vi "Set Resistor copy.vi"(8 "error in":errorcluster, 9 "Set Resistance":T1) -> (0 "error out":errorcluster)   [LabVIEW 2019]
uses:
  <userlib>/LevyLab/Relay Box/Relay-Box.lvclass
  <userlib>/LevyLab/Relay Box/subVIs/Control Relay (256).vi
  <userlib>/LevyLab/Relay Box/Typedefs/Resistor--enum.ctl
panel:
  out "USB":bool
  out "short":bool
  out "0 ohm":bool
  out "100k":bool
  out "10M":bool
  out "Gohm":bool
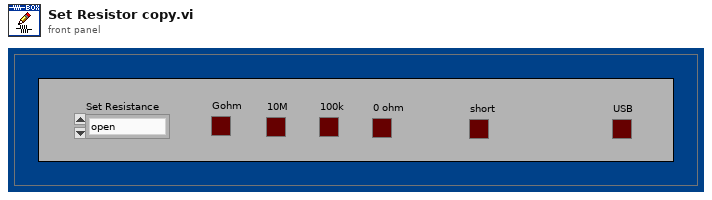
[diagram p1: front panel]
types:
  T1 = typedef "Resistor--enum.ctl" = enum16{"open", "discharge tip", "0 ohms", "100k ohm", "10M ohm", "1G ohm"}
  T2 = enum32{"Invalid", "Standard", "Closed", "Hidden", "Minimized", "Maximized"}
  T3 = enum32{"invalid app kind", "Development System", "Run Time System", "Student Edition", "Embedded LabVIEW", "Evaluation", "Custom"}
  T4 = cluster{"Core":cluster{"Current VI Reference":refnum<vi>, "Close Panel on Exit?":bool}, "Set Resistance":T1, "Previous State":u8, "Intermediate State":u8, "Final State":u8, "Bool Status":bool[]}
  T5 = cluster{"Current VI Reference":refnum<vi>, "Close Panel on Exit?":bool}
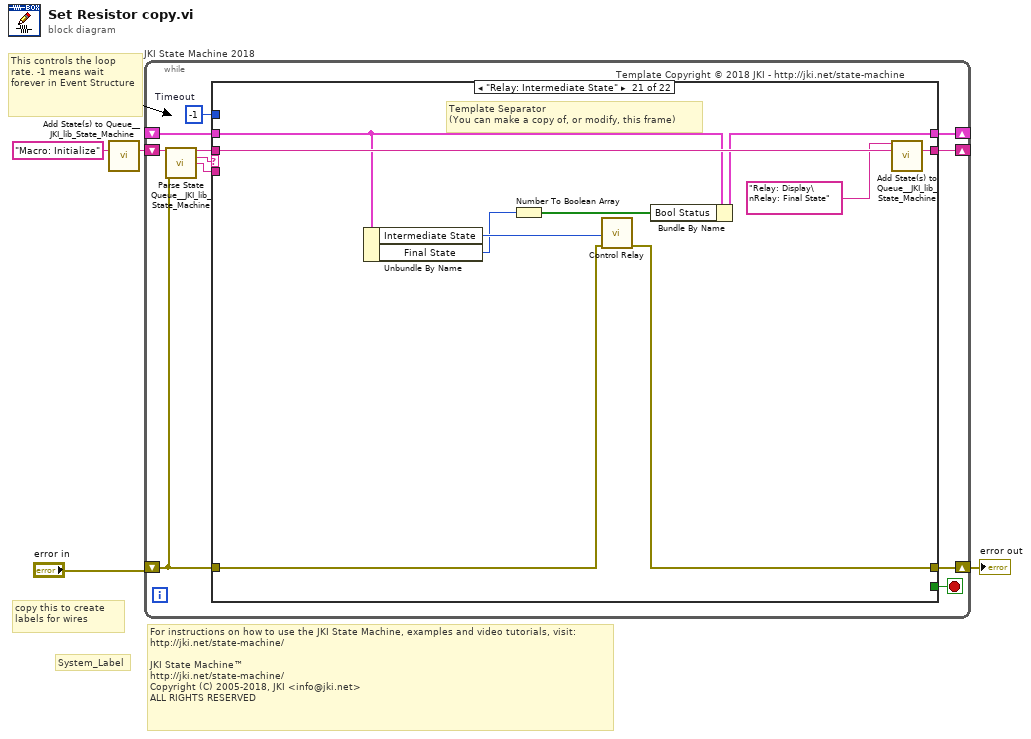
[diagram p0: block diagram]
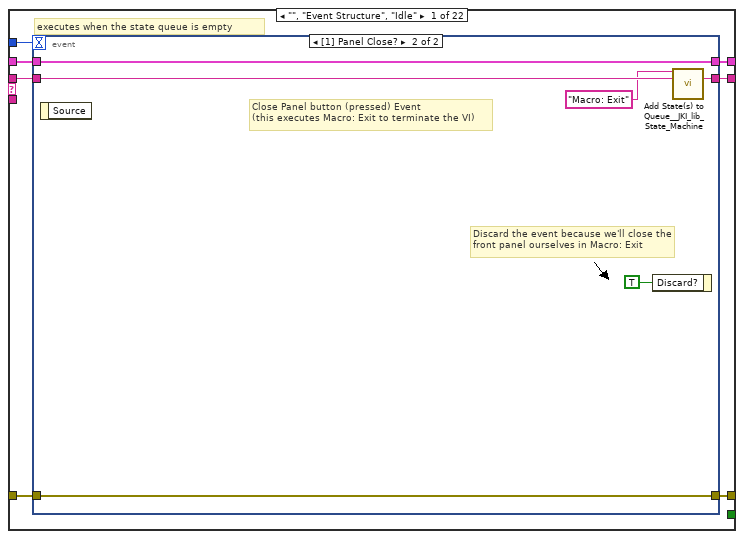
[diagram p2: hidden frame]
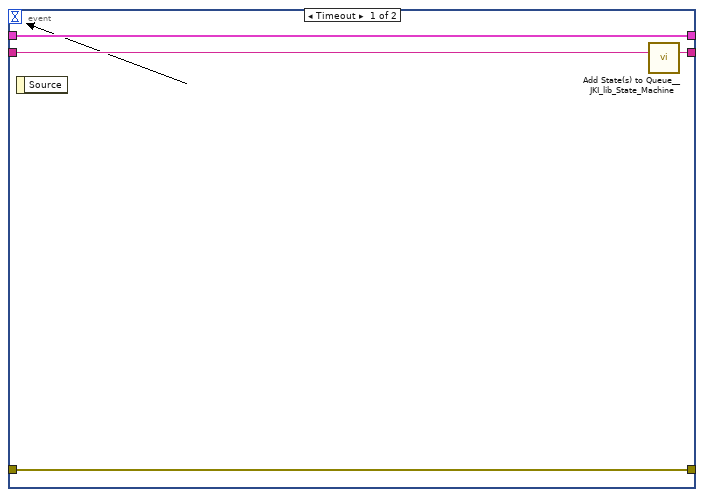
[diagram p3: hidden frame]
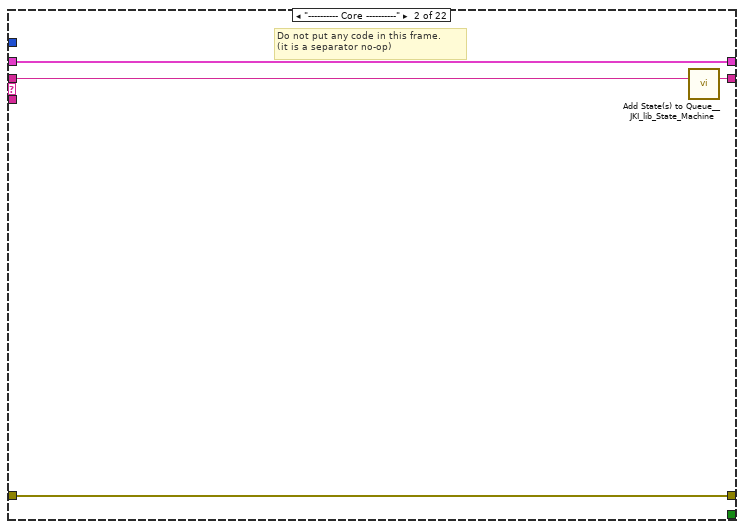
[diagram p4: hidden frame]
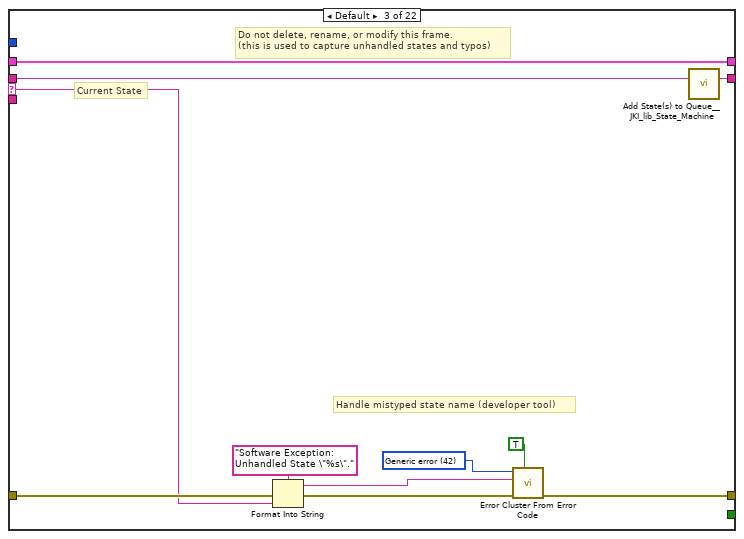
[diagram p5: hidden frame]
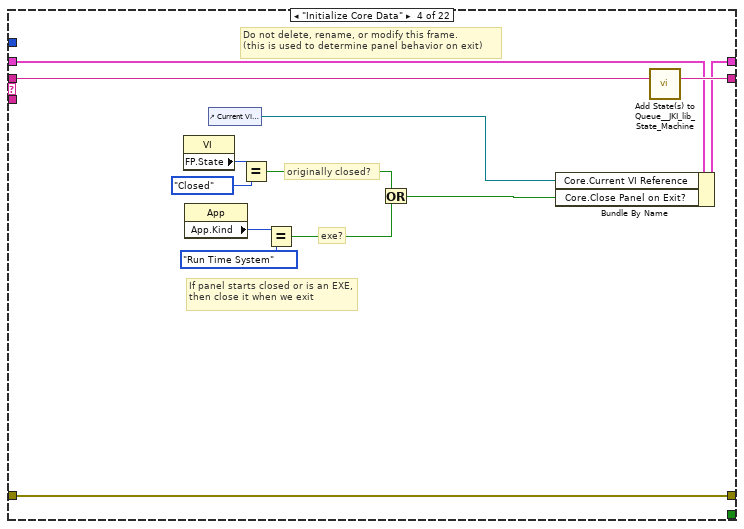
[diagram p6: hidden frame]
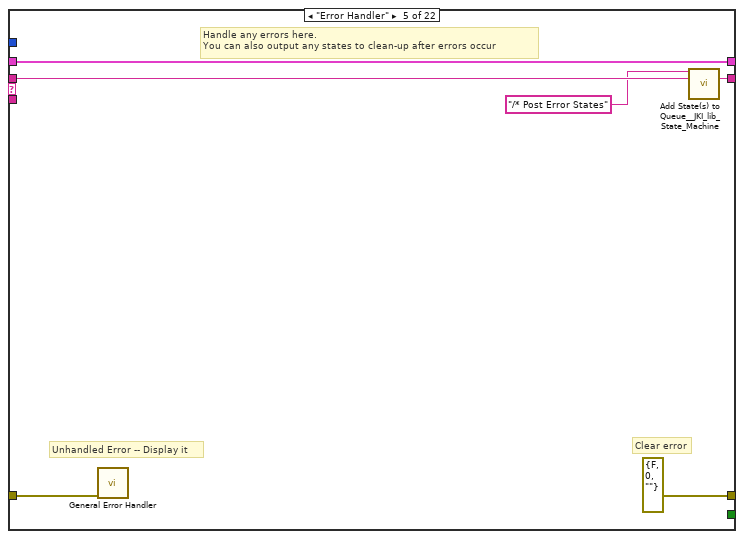
[diagram p7: hidden frame]
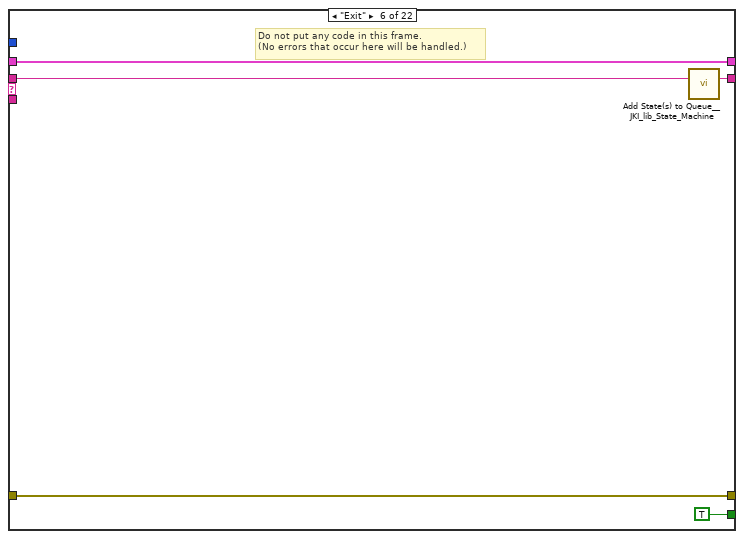
[diagram p8: hidden frame]
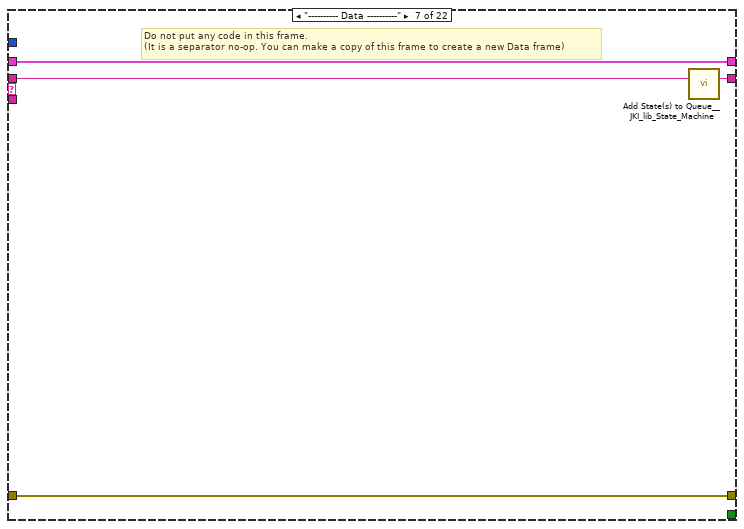
[diagram p9: hidden frame]
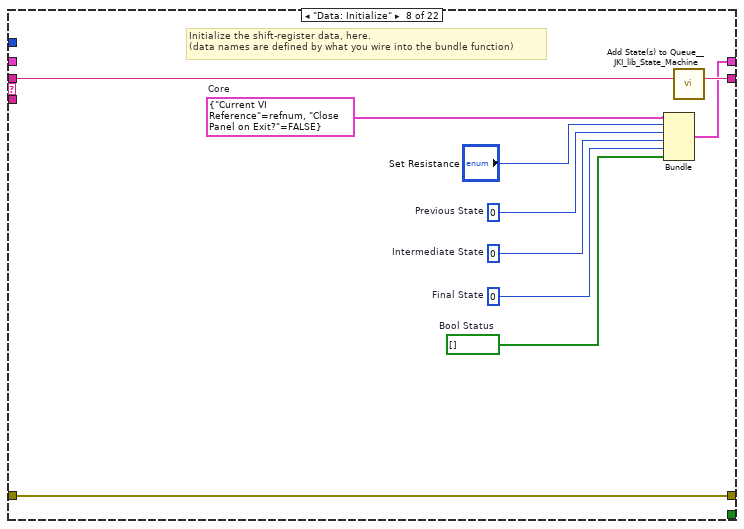
[diagram p10: hidden frame]
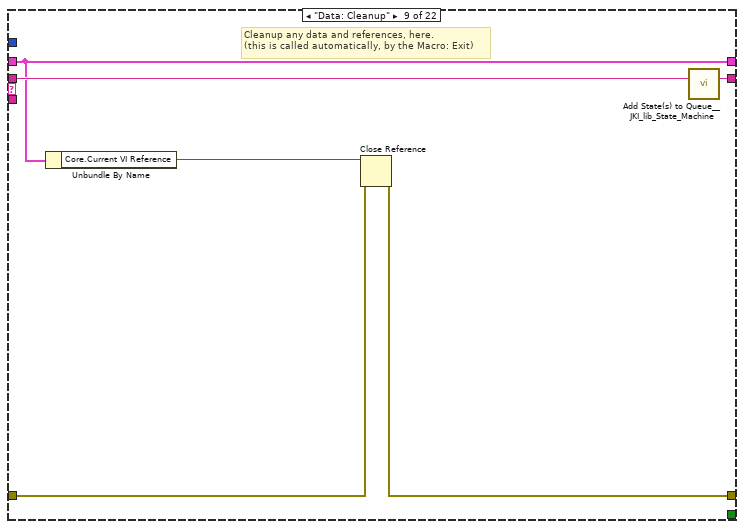
[diagram p11: hidden frame]
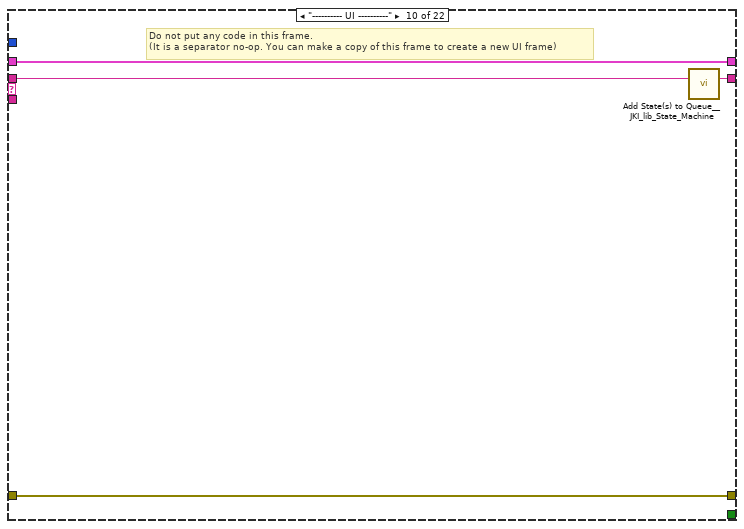
[diagram p12: hidden frame]
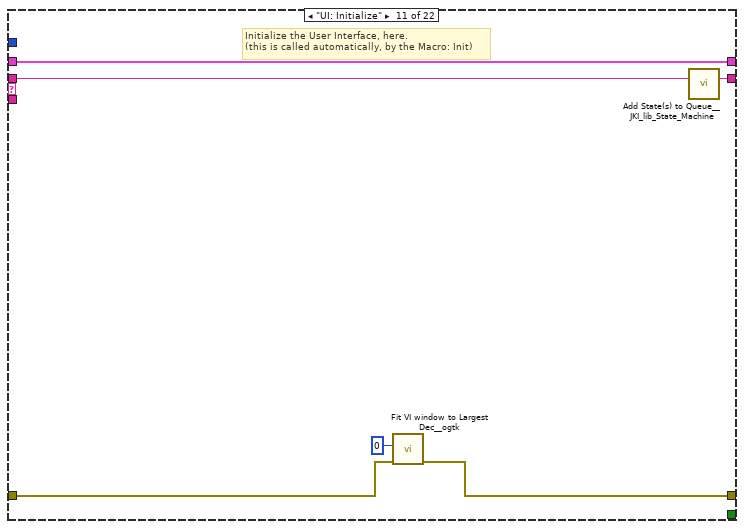
[diagram p13: hidden frame]
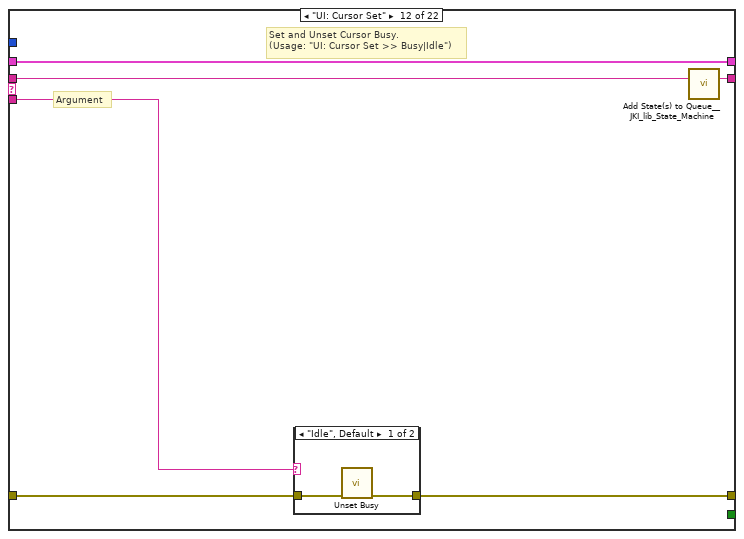
[diagram p14: hidden frame]
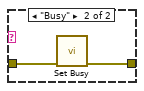
[diagram p15: hidden frame]
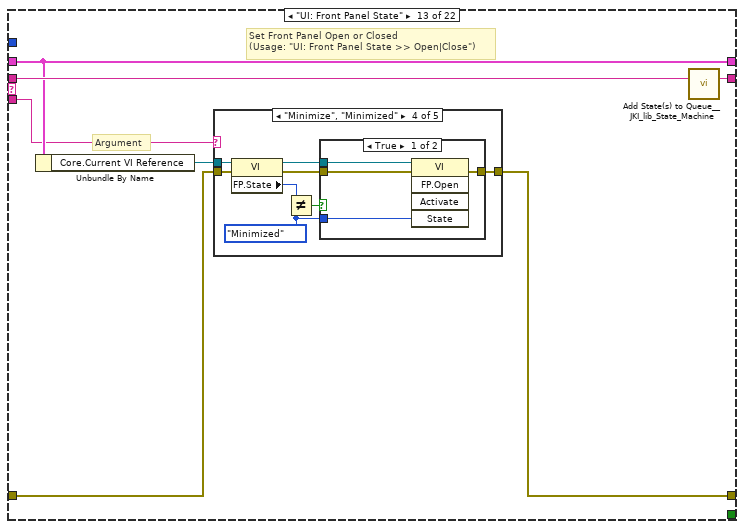
[diagram p16: hidden frame]
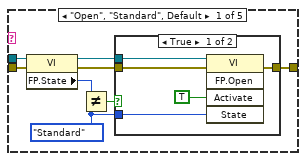
[diagram p17: hidden frame]
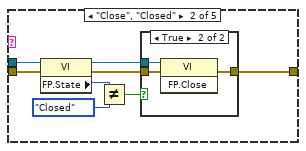
[diagram p19: hidden frame]
diagram:
  # "For instructions on how to use the JKI State Machine, examples and video tutorials, visit:\nhttp://jki.net/state-machine/\n\nJKI State Machine™\nhttp://jki.net/state-machine/\nCopyright (C) 2005-2018, JKI <info@jki.net>\nALL RIGHTS RESERVED"
  # "copy this to create labels for wires"
  # "This controls the loop rate. -1 means wait forever in Event Structure"
  # "System_Label"
  n1 = call <vilib>:"Add State(s) to Queue__JKI_lib_State_Machine.vi"("State(s) in (\"\")"="Macro: Initialize") -> ("States Out"=w4:string)  [unwired: 14 in]
  n2 = while "JKI State Machine 2018" {
    shift-right: [w8] -> _
    shift-left: _ -> [w7]
    shift-right: [w11] -> w2
    shift-left: "error in" -> [w5]
    shift-right: [w10] -> _
    shift-left: w4 -> [w12]
    stop <- w9 stop-if-true
    w6 = -1  # Timeout
    # "Template Copyright © 2018 JKI - http://jki.net/state-machine"
    n3 = call <vilib>:"Parse State Queue__JKI_lib_State_Machine.vi"("State Queue"=w12, "Error In (no error)"=w5) -> ("Remaining States"=w14:string, "Current State"=w15:string, "Arguments"=w13:string)  [unwired: 11 in]
    n4 = case shown="\"Relay: Intermediate State\"" w15 {
      selector: w15 -> [_ _ w37 _ _ _ _ _ _ _ _ _ _ _ _ _ _ _ _ _ _ _]
      tunnel: w14 -> [w22 w36 w41 w60 w66 w71 w75 w85 w91 w95 w101 w107 w118 w187 w192 w202 w206 w222 w230 w244 w368 w375]
      tunnel: w13 -> [_ _ _ _ _ _ _ _ _ _ _ w102 w112 _ _ _ _ _ _ _ _ _]
      tunnel: w7 -> [w20 w33 w39 w53 w63 w69 w72 _ w86 w92 w99 w105 w114 w184 w189 w199 w203 w216 w225 w233 w361 w369]
      tunnel: [w19 w34 w43 w57 errorcluster {"status"=FALSE, "code"=0, "source"=""} ("error out") w68 w73 w83 w87 w93 w97 w103 w115 w185 w190 w200 w204 w220 w228 w242 w362 w371] -> w11
      tunnel: w5 -> [w18 w34 w42 w57 w62 w68 w73 w83 w88 w93 w96 w104 w116 w185 w190 w200 w204 w220 w228 w242 w363 w372]
      tunnel: [w21 w35 w40 w59 w65 w70 w74 w84 w90 w94 w100 w106 w117 w186 w191 w201 w205 w221 w229 w243 w367 w374] -> w10
      tunnel: [_ _ _ _ _ TRUE _ _ _ _ _ _ _ _ _ _ _ _ _ _ _ _] -> w9
      tunnel: [w17 w33 w39 w58 w63 w69 w72 w77 w86 w92 w99 w105 w114 w184 w189 w199 w203 w216 w224 w232 w360 w369] -> w8
      tunnel: w6 -> [w16 _ _ _ _ _ _ _ _ _ _ _ _ _ _ _ _ _ _ _ _ _]
      frame "", "Event Structure", "Idle" {
        # "executes when the state queue is empty"
        n5 = event shown="[1] Panel Close?" {
          selector: _ -> [_ _]
          dyn-events: _ -> [_ _]
          timeout: w16 -> [_ _]
          tunnel: w22 -> [w26 w32]
          tunnel: [w25 w31] -> w21
          tunnel: w20 -> [w23 w29]
          tunnel: [w24 w30] -> w19
          tunnel: w18 -> [w24 w30]
          tunnel: [w23 w29] -> w17
          event Timeout {
            n6 = event-data() -> ()  [unwired: 1 in, 1 out]
            n7 = call <vilib>:"Add State(s) to Queue__JKI_lib_State_Machine.vi"("State(s) in (\"\")"=w26) -> ("States Out"=w25:string)  [unwired: 14 in]
          }
          event Panel Close? {
            # "Discard the event because we'll close the front panel ourselves in Macro: Exit"
            # "Close Panel button (pressed) Event\n(this executes Macro: Exit to terminate the VI)"
            n8 = event-data() -> ()  [unwired: 1 in, 1 out]
            n9 = event-data("Discard?"=TRUE) -> ()  [unwired: 1 in, 1 out]
            n10 = call <vilib>:"Add State(s) to Queue__JKI_lib_State_Machine.vi"("State(s) in Front (\"\")"="Macro: Exit", "State(s) in (\"\")"=w32) -> ("States Out"=w31:string)  [unwired: 13 in]
          }
        }
      }
      frame "---------- Core ----------" {
        # "Do not put any code in this frame.\n(it is a separator no-op)"
        n11 = call <vilib>:"Add State(s) to Queue__JKI_lib_State_Machine.vi"("State(s) in (\"\")"=w36) -> ("States Out"=w35:string)  [unwired: 14 in]
      }
      frame Default {
        w46 = 42 items=["No error", "Argument error", "Memory is full", "Out of zone", "End of file", "File already open", "Generic file I/O error", "File not found", "File permission error", "Disk is full", "Duplicate path", "Too many files open", "System feature not enabled", "Resource file not found", "Cannot add resource", "Resource not found", "Image not found", "Image memory error", "Pen does not exist", "Config type invalid", "Config token not found", "Config parse error", "Config memory error", "Bad external code format", "Bad external code offset", "External code not present", "Null window", "Destroy window error", "Null menu", "Print aborted", "Bad print record", "Print driver error", "Windows error during printing", "Memory error during printing", "Print dialog error", "Generic print error", "Invalid device refnum", "Device not found", "Device parameter error", "Device unit error", "Cannot open device", "Device call aborted", "Generic error", "Cancelled by user", "Object ID too low", "Object ID too high", "Object not in heap", "Unknown heap", "Unknown object (invalid DefProc)", "Unknown object (DefProc not in table)", "Message out of range", "Invalid (null) method", "Unknown message", "Manager call not supported", "Bad address", "Network operation in progress", "Network operation timed out", "Connection is busy", "Network attribute not supported", "Network error", "Address in use", "System out of memory", "Connection aborted", "Connection refused", "Not connected", "Already connected", "Connection closed", "Initialization error (interapplication manager)", "Bad occurrence", "Wait on unbound occurrence handler", "Occurrence queue overflow", "Datalog type conflict", "Unused", "Unrecognized type (interapplication manager)", "Memory corrupt", "Failed to make temporary DLL", "Old CIN version", "Drag socket not found", "Failed to load drop-object", "Failed to register OLE object", "Failed to release OLE object", "Format specifier type mismatch", "Unknown format specifier", "Too few format specifiers", "Too many format specifiers", "Scan failed", "Newer CIN version", "Error converting to variant", "Runtime menu error", "Password tampered", "Variant attribute not found", "Incompatible variant data type", "Event data is not available", "Event Store is not present", "Occurrence is not found", "Event Queue is not created", "Event info is not available", "Refnum passed is NULL", "Error retrieving Class GUID", "Error retrieving CoClass GUID", "Error retrieving TypeLib GUID.", "Bad built application magic bytes.", "Specific driver is different from the specific driver associated with the Logical Name.", "There is no session opened to the class driver.", "Max Error", "MAX - Error with config objects", "MAX - Error loading configuration", "MAX - Group not supported"]
        # "Current State"
        # "Do not delete, rename, or modify this frame.\n(this is used to capture unhandled states and typos)"
        # "Handle mistyped state name (developer tool)"
        n12 = Format Into String(format string="Software Exception: Unhandled State \"%s\"." ("message"), error in=w42, w37) -> (resulting string=w45:string, error out=w44:errorcluster)  [unwired: 1 in]
        n13 = call <vilib>:"Error Cluster From Error Code.vi"("show call chain? (False)"=TRUE, "error in (no error)"=w44, "error message (\"\")"=w45, "error code (0)"=w46) -> ("error out"=w43:errorcluster)  [unwired: 5 in]
        n14 = call <vilib>:"Add State(s) to Queue__JKI_lib_State_Machine.vi"("State(s) in (\"\")"=w41) -> ("States Out"=w40:string)  [unwired: 14 in]
      }
      frame "Initialize Core Data" {
        # "Do not delete, rename, or modify this frame.\n(this is used to determine panel behavior on exit)"
        # "originally closed?"
        # "exe?"
        # "If panel starts closed or is an EXE, then close it when we exit"
        n15 = property class="VI"() -> ("FP.State"=w50:T2)  [unwired: 2 in, 2 out]
        n16 = property class="App"() -> ("App.Kind"=w56:T3)  [unwired: 2 in, 2 out]
        n17 = control-ref of="Current VI Reference"() -> (w51:refnum<vi>)
        n18 = Equal?(x=w50, y=T2."Closed" ("Front Panel Window:State")) -> (x = y?=w48:bool)
        n19 = Equal?(x=w56, y=T3."Run Time System" ("Application:Kind")) -> (x = y?=w54:bool)
        n20 = Or(x=w48, y=w54) -> (x .or. y?=w52:bool)
        n21 = Bundle By Name(cluster=w53, "Core.Current VI Reference"=w51, "Core.Close Panel on Exit?"=w52) -> (w58:T4)
        n22 = call <vilib>:"Add State(s) to Queue__JKI_lib_State_Machine.vi"("State(s) in (\"\")"=w60) -> ("States Out"=w59:string)  [unwired: 14 in]
      }
      frame "Error Handler" {
        # "Unhandled Error -- Display it"
        # "Handle any errors here.\nYou can also output any states to clean-up after errors occur"
        # "Clear error"
        n23 = call <vilib>:"General Error Handler.vi"("error in (no error)"=w62) -> ()  [unwired: 10 in, 5 out]
        n24 = call <vilib>:"Add State(s) to Queue__JKI_lib_State_Machine.vi"("State(s) in Front (\"\")"="/* Post Error States", "State(s) in (\"\")"=w66) -> ("States Out"=w65:string)  [unwired: 13 in]
      }
      frame "Exit" {
        # "Do not put any code in this frame.\n(No errors that occur here will be handled.)"
        n25 = call <vilib>:"Add State(s) to Queue__JKI_lib_State_Machine.vi"("State(s) in (\"\")"=w71) -> ("States Out"=w70:string)  [unwired: 14 in]
      }
      frame "---------- Data ----------" {
        # "Do not put any code in this frame.\n(It is a separator no-op. You can make a copy of this frame to create a new Data frame)"
        n26 = call <vilib>:"Add State(s) to Queue__JKI_lib_State_Machine.vi"("State(s) in (\"\")"=w75) -> ("States Out"=w74:string)  [unwired: 14 in]
      }
      frame "Data: Initialize" {
        w76 = bool[] []  # Bool Status
        w79 = u8 0  # Final State
        w80 = u8 0  # Intermediate State
        w81 = u8 0  # Previous State
        w78 = T5 {"Current VI Reference"=refnum, "Close Panel on Exit?"=FALSE}  # Core
        # "Initialize the shift-register data, here.\n(data names are defined by what you wire into the bundle function)"
        n27 = Bundle("Core"=w78, "Set Resistance"="Set Resistance", "Previous State"=w81, "Intermediate State"=w80, "Final State"=w79, "Bool Status"=w76) -> (w77:T4)  [unwired: 1 in]
        n28 = call <vilib>:"Add State(s) to Queue__JKI_lib_State_Machine.vi"("State(s) in (\"\")"=w85) -> ("States Out"=w84:string)  [unwired: 14 in]
      }
      frame "Data: Cleanup" {
        # "Cleanup any data and references, here.\n(this is called automatically, by the Macro: Exit)"
        n29 = Unbundle By Name(w86) -> ("Core.Current VI Reference"=w89:refnum<vi>)
        n30 = Close Reference(reference=w89, error in (no error)=w88) -> (error out=w87:errorcluster)
        n31 = call <vilib>:"Add State(s) to Queue__JKI_lib_State_Machine.vi"("State(s) in (\"\")"=w91) -> ("States Out"=w90:string)  [unwired: 14 in]
      }
      frame "---------- UI ----------" {
        # "Do not put any code in this frame.\n(It is a separator no-op. You can make a copy of this frame to create a new UI frame)"
        n32 = call <vilib>:"Add State(s) to Queue__JKI_lib_State_Machine.vi"("State(s) in (\"\")"=w95) -> ("States Out"=w94:string)  [unwired: 14 in]
      }
      frame "UI: Initialize" {
        # "Initialize the User Interface, here.\n(this is called automatically, by the Macro: Init)"
        n33 = call <userlib>:"Fit VI window to Largest Dec__ogtk.vi"("error in (no error)"=w96, "border spacing (2 px)"=0) -> ("error out"=w97:errorcluster)  [unwired: 4 in, 1 out]
        n34 = call <vilib>:"Add State(s) to Queue__JKI_lib_State_Machine.vi"("State(s) in (\"\")"=w101) -> ("States Out"=w100:string)  [unwired: 14 in]
      }
      frame "UI: Cursor Set" {
        # "Argument"
        # "Set and Unset Cursor Busy.\n(Usage: \"UI: Cursor Set >> Busy|Idle\")"
        n35 = case shown="\"Idle\", Default" w102 {
          tunnel: w104 -> [w109 w111]
          tunnel: [w108 w110] -> w103
          frame "Idle", Default {
            n36 = call <vilib>:"Unset Busy.vi"("error in (no error)"=w109) -> ("error out"=w108:errorcluster)  [unwired: 10 in]
          }
          frame "Busy" {
            n37 = call <vilib>:"Set Busy.vi"("error in (no error)"=w111) -> ("error out"=w110:errorcluster)  [unwired: 9 in, 1 out]
          }
        }
        n38 = call <vilib>:"Add State(s) to Queue__JKI_lib_State_Machine.vi"("State(s) in (\"\")"=w107) -> ("States Out"=w106:string)  [unwired: 14 in]
      }
      frame "UI: Front Panel State" {
        # "Argument"
        # "Set Front Panel Open or Closed\n(Usage: \"UI: Front Panel State >> Open|Close\")"
        n39 = Unbundle By Name(w114) -> ("Core.Current VI Reference"=w113:refnum<vi>)
        n40 = case shown="\"Minimize\", \"Minimized\"" w112 {
          tunnel: w116 -> [w124 w139 w150 w163 w176]
          tunnel: [w126 w140 w152 w165 w178] -> w115
          tunnel: w113 -> [w125 w137 w151 w164 w177]
          frame "Open", "Standard", Default {
            w119 = T2."Standard" ("State")
            n41 = property class="VI"(reference=w125, error in=w124) -> (reference out=w122:refnum<vi>, error out=w123:errorcluster, "FP.State"=w121:T2)
            n42 = Not Equal?(x=w121, y=w119) -> (x != y?=w120:bool)
            n43 = case shown="True" w120 {
              tunnel: [w130 w132] -> w126
              tunnel: w123 -> [w129 w132]
              tunnel: w122 -> [w128 _]
              tunnel: w119 -> [w127 _]
              frame True {
                n44 = invoke class="VI" method="FP.Open"(reference=w128, error in=w129, "Activate"=TRUE, "State"=w127) -> (error out=w130:errorcluster)  [unwired: 1 in, 4 out]
              }
              frame False {
              }
            }
          }
          frame "Close", "Closed" {
            n45 = property class="VI"(reference=w137, error in=w139) -> (reference out=w136:refnum<vi>, error out=w138:errorcluster, "FP.State"=w134:T2)
            n46 = Not Equal?(x=w134, y=T2."Closed" ("Front Panel Window:State")) -> (x != y?=w133:bool)
            n47 = case shown="True" w133 {
              tunnel: [w141 w144] -> w140
              tunnel: w138 -> [w141 w143]
              tunnel: w136 -> [_ w142]
              frame False {
              }
              frame True {
                n48 = invoke class="VI" method="FP.Close"(reference=w142, error in=w143) -> (error out=w144:errorcluster)  [unwired: 1 in, 2 out]
              }
            }
          }
          frame "Hidden", "Hide" {
            w145 = T2."Hidden" ("State")
            n49 = property class="VI"(reference=w151, error in=w150) -> (reference out=w148:refnum<vi>, error out=w149:errorcluster, "FP.State"=w147:T2)
            n50 = Not Equal?(x=w147, y=w145) -> (x != y?=w146:bool)
            n51 = case shown="True" w146 {
              tunnel: [w156 w157] -> w152
              tunnel: w149 -> [w155 w157]
              tunnel: w148 -> [w154 _]
              tunnel: w145 -> [w153 _]
              frame True {
                n52 = invoke class="VI" method="FP.Open"(reference=w154, error in=w155, "State"=w153) -> (error out=w156:errorcluster)  [unwired: 2 in, 4 out]
              }
              frame False {
              }
            }
          }
          frame "Minimize", "Minimized" {
            w158 = T2."Minimized" ("State")
            n53 = property class="VI"(reference=w164, error in=w163) -> (reference out=w161:refnum<vi>, error out=w162:errorcluster, "FP.State"=w160:T2)
            n54 = Not Equal?(x=w160, y=w158) -> (x != y?=w159:bool)
            n55 = case shown="True" w159 {
              tunnel: [w169 w170] -> w165
              tunnel: w162 -> [w168 w170]
              tunnel: w161 -> [w167 _]
              tunnel: w158 -> [w166 _]
              frame True {
                n56 = invoke class="VI" method="FP.Open"(reference=w167, error in=w168, "State"=w166) -> (error out=w169:errorcluster)  [unwired: 2 in, 4 out]
              }
              frame False {
              }
            }
          }
          frame "Maximize", "Maximized" {
            w171 = T2."Maximized" ("State")
            n57 = property class="VI"(reference=w177, error in=w176) -> (reference out=w174:refnum<vi>, error out=w175:errorcluster, "FP.State"=w173:T2)
            n58 = Not Equal?(x=w173, y=w171) -> (x != y?=w172:bool)
            n59 = case shown="True" w172 {
              tunnel: [w182 w183] -> w178
              tunnel: w175 -> [w181 w183]
              tunnel: w174 -> [w180 _]
              tunnel: w171 -> [w179 _]
              frame True {
                n60 = invoke class="VI" method="FP.Open"(reference=w180, error in=w181, "State"=w179) -> (error out=w182:errorcluster)  [unwired: 2 in, 4 out]
              }
              frame False {
              }
            }
          }
        }
        n61 = call <vilib>:"Add State(s) to Queue__JKI_lib_State_Machine.vi"("State(s) in (\"\")"=w118) -> ("States Out"=w117:string)  [unwired: 14 in]
      }
      frame "---------- Macro ----------" {
        # "Do not put any code in this frame.\n(It is a separator no-op. You can make a copy of this frame to create a new Macro frame)"
        n62 = call <vilib>:"Add State(s) to Queue__JKI_lib_State_Machine.vi"("State(s) in (\"\")"=w187) -> ("States Out"=w186:string)  [unwired: 14 in]
      }
      frame "Macro: Initialize" {
        # "Initialization Macro\n(This is called once, when the VI starts)"
        n63 = call <vilib>:"Add State(s) to Queue__JKI_lib_State_Machine.vi"("State(s) in Front (\"\")"="Data: Initialize\nInitialize Core Data\nUI: Initialize\nRelay: Read\nRelay: Do Logic", "State(s) in (\"\")"=w192) -> ("States Out"=w191:string)  [unwired: 13 in]
      }
      frame "Macro: Exit" {
        # "Exit Macro\n(This is called once, when the VI exits)"
        n64 = Unbundle By Name(w199) -> ("Core.Close Panel on Exit?"=w198:bool)
        n65 = Select(t="UI: Front Panel State >> Close", s=w198, f="") -> (s? t:f=w195:string)
        n66 = call <vilib>:"Add State(s) to Queue__JKI_lib_State_Machine.vi"("State(s) in (\"\")"=w195, "State(s) at Back (\"\")"="Data: Cleanup\nExit") -> ("States Out"=w193:string)  [unwired: 13 in]
        n67 = call <vilib>:"Add State(s) to Queue__JKI_lib_State_Machine.vi"("State(s) in Front (\"\")"=w193, "State(s) in (\"\")"=w202) -> ("States Out"=w201:string)  [unwired: 13 in]
      }
      frame "---------- Relay ----------" {
        # "Template Separator\n(You can make a copy of, or modify, this frame)"
        n68 = call <vilib>:"Add State(s) to Queue__JKI_lib_State_Machine.vi"("State(s) in (\"\")"=w206) -> ("States Out"=w205:string)  [unwired: 14 in]
      }
      frame "Relay: Display" {
        # "Your code here.\n(You can make a copy of, or modify, this frame)"
        n69 = Unbundle By Name(w216) -> ("Bool Status"=w215:bool[])
        n70 = Index Array(array=w215, index #1=7 ("index"), index #2=6 ("index"), index #3=5 ("index"), index #4=3 ("index"), index #5=1 ("index")) -> (element #1=→"Gohm":bool, element #2=→"10M":bool, element #3=→"100k":bool, element #4=→"0 ohm":bool, element #5=→"short":bool)
        n71 = call <vilib>:"Add State(s) to Queue__JKI_lib_State_Machine.vi"("State(s) in (\"\")"=w222) -> ("States Out"=w221:string)  [unwired: 14 in]
        "USB" <- TRUE ("USB")
      }
      frame "Relay: Read" {
        # "Your code here.\n(You can make a copy of, or modify, this frame)"
        n72 = call <userlib>:"Read Relay.vi"() -> ("unsigned 8bit integer"=w227:u8, "Boolean array"=w226:bool[])  [unwired: 1 in]
        n73 = Bundle By Name(cluster=w225, "Previous State"=w227, "Bool Status"=w226) -> (w224:T4)
        n74 = call <vilib>:"Add State(s) to Queue__JKI_lib_State_Machine.vi"("State(s) in Front (\"\")"="Relay: Display" ("State(s) in Front (\"\")"), "State(s) in (\"\")"=w230) -> ("States Out"=w229:string)  [unwired: 13 in]
      }
      frame "Relay: Do Logic" {
        # "Template Separator\n(You can make a copy of, or modify, this frame)"
        n75 = Unbundle By Name(w233) -> ("Set Resistance"=w241:T1, "Previous State"=w237:u8)
        n76 = case shown="\"0 ohms\"" w241 {
          tunnel: [u8 0 w248 w256 w282 w308 w334] -> w236
          tunnel: [FALSE w249 w255 w281 w307 w333] -> w231
          tunnel: [0 2 8 32 64 128] -> w238
          tunnel: w237 -> [_ w251 w257 w283 w309 w335]
          frame "open", Default {
          }
          frame "discharge tip" {
            n77 = Not Equal?(x=w251, y=u8 0) -> (x != y?=w249:bool)
            n78 = case shown="True" w249 {
              tunnel: [u8 2 u8 0] -> w248
              frame False {
              }
              frame True {
              }
            }
          }
          frame "0 ohms" {
            n79 = Not Equal?(x=w257, y=u8 2) -> (x != y?=w258:bool)
            n80 = case shown="True" w258 {
              tunnel: w257 -> [_ w265]
              tunnel: [u8 0 w264] -> w256
              tunnel: [TRUE w263] -> w255
              frame False {
              }
              frame True {
                n81 = Not Equal?(x=w265, y=u8 0) -> (x != y?=w266:bool)
                n82 = case shown="True" w266 {
                  tunnel: w265 -> [_ w273]
                  tunnel: [u8 8 w271] -> w264
                  tunnel: [FALSE w270] -> w263
                  frame False {
                  }
                  frame True {
                    w272 = u8 8 ("y")
                    n83 = Not Equal?(x=w273, y=w272) -> (x != y?=w274:bool)
                    n84 = case shown="False" w274 {
                      tunnel: w273 -> [_ w280]
                      tunnel: w272 -> [_ w279]
                      tunnel: [u8 8 w278] -> w271
                      tunnel: [FALSE TRUE] -> w270
                      frame False {
                      }
                      frame True {
                        n85 = Add(x=w280, y=w279) -> (x+y=w278:u8)
                      }
                    }
                  }
                }
              }
            }
          }
          frame "100k ohm" {
            n86 = Not Equal?(x=w283, y=u8 2) -> (x != y?=w284:bool)
            n87 = case shown="True" w284 {
              tunnel: w283 -> [_ w291]
              tunnel: [u8 0 w290] -> w282
              tunnel: [TRUE w289] -> w281
              frame False {
              }
              frame True {
                n88 = Not Equal?(x=w291, y=u8 0) -> (x != y?=w292:bool)
                n89 = case shown="False" w292 {
                  tunnel: w291 -> [_ w299]
                  tunnel: [u8 32 w297] -> w290
                  tunnel: [FALSE w296] -> w289
                  frame False {
                  }
                  frame True {
                    w298 = u8 32 ("y")
                    n90 = Not Equal?(x=w299, y=w298) -> (x != y?=w300:bool)
                    n91 = case shown="True" w300 {
                      tunnel: w299 -> [_ w306]
                      tunnel: w298 -> [_ w305]
                      tunnel: [u8 32 w304] -> w297
                      tunnel: [FALSE TRUE] -> w296
                      frame False {
                      }
                      frame True {
                        n92 = Add(x=w306, y=w305) -> (x+y=w304:u8)
                      }
                    }
                  }
                }
              }
            }
          }
          frame "10M ohm" {
            n93 = Not Equal?(x=w309, y=u8 2) -> (x != y?=w310:bool)
            n94 = case shown="True" w310 {
              tunnel: w309 -> [_ w317]
              tunnel: [u8 0 w316] -> w308
              tunnel: [TRUE w315] -> w307
              frame False {
              }
              frame True {
                n95 = Not Equal?(x=w317, y=u8 0) -> (x != y?=w318:bool)
                n96 = case shown="False" w318 {
                  tunnel: w317 -> [_ w325]
                  tunnel: [u8 64 w323] -> w316
                  tunnel: [FALSE w322] -> w315
                  frame False {
                  }
                  frame True {
                    w324 = u8 64 ("y")
                    n97 = Not Equal?(x=w325, y=w324) -> (x != y?=w326:bool)
                    n98 = case shown="False" w326 {
                      tunnel: w325 -> [_ w332]
                      tunnel: w324 -> [_ w331]
                      tunnel: [u8 64 w330] -> w323
                      tunnel: [FALSE TRUE] -> w322
                      frame False {
                      }
                      frame True {
                        n99 = Add(x=w332, y=w331) -> (x+y=w330:u8)
                      }
                    }
                  }
                }
              }
            }
          }
          frame "1G ohm" {
            n100 = Not Equal?(x=w335, y=u8 2) -> (x != y?=w336:bool)
            n101 = case shown="True" w336 {
              tunnel: w335 -> [_ w343]
              tunnel: [u8 0 w342] -> w334
              tunnel: [TRUE w341] -> w333
              frame False {
              }
              frame True {
                n102 = Not Equal?(x=w343, y=u8 0) -> (x != y?=w344:bool)
                n103 = case shown="False" w344 {
                  tunnel: w343 -> [_ w351]
                  tunnel: [u8 128 w349] -> w342
                  tunnel: [FALSE w348] -> w341
                  frame False {
                  }
                  frame True {
                    w350 = u8 128 ("y")
                    n104 = Not Equal?(x=w351, y=w350) -> (x != y?=w352:bool)
                    n105 = case shown="True" w352 {
                      tunnel: w351 -> [_ w358]
                      tunnel: w350 -> [_ w357]
                      tunnel: [u8 128 w356] -> w349
                      tunnel: [FALSE TRUE] -> w348
                      frame False {
                      }
                      frame True {
                        n106 = Add(x=w358, y=w357) -> (x+y=w356:u8)
                      }
                    }
                  }
                }
              }
            }
          }
        }
        n107 = Number To Boolean Array(number=w236) -> (Boolean array=w235:bool[])
        n108 = Bundle By Name(cluster=w233, "Bool Status"=w235, "Intermediate State"=w236, "Final State"=w238) -> (w232:T4)
        n109 = Select(t="Relay: Display\nRelay: Intermediate State", s=w231, f="Relay: Display\nRelay: Final State") -> (s? t:f=w234:string)
        n110 = call <vilib>:"Add State(s) to Queue__JKI_lib_State_Machine.vi"("State(s) in Front (\"\")"=w234, "State(s) in (\"\")"=w244) -> ("States Out"=w243:string)  [unwired: 13 in]
      }
      frame "Relay: Intermediate State" {
        # "Template Separator\n(You can make a copy of, or modify, this frame)"
        n111 = Unbundle By Name(w361) -> ("Intermediate State"=w365:u8, "Final State"=w364:u8)
        n112 = Number To Boolean Array(number=w364) -> (Boolean array=w366:bool[])
        n113 = call-poly <userlib>:"Control Relay.vi"("error in (no error)"=w363, "Send to relay board"=w365) -> ("error out"=w362:errorcluster)  [unwired: 9 in]
        n114 = Bundle By Name(cluster=w361, "Bool Status"=w366) -> (w360:T4)
        n115 = call <vilib>:"Add State(s) to Queue__JKI_lib_State_Machine.vi"("State(s) in Front (\"\")"="Relay: Display\nRelay: Final State" ("State(s) in Front (\"\")"), "State(s) in (\"\")"=w368) -> ("States Out"=w367:string)  [unwired: 13 in]
      }
      frame "Relay: Final State" {
        # "Template Separator\n(You can make a copy of, or modify, this frame)"
        n116 = Unbundle By Name(w369) -> ("Final State"=w373:u8)
        n117 = call-poly <userlib>:"Control Relay.vi"("error in (no error)"=w372, "Send to relay board"=w373) -> ("error out"=w371:errorcluster)  [unwired: 9 in]
        n118 = call <vilib>:"Add State(s) to Queue__JKI_lib_State_Machine.vi"("State(s) in Front (\"\")"="Relay: Read\nMacro: Exit" ("State(s) in Front (\"\")"), "State(s) in (\"\")"=w375) -> ("States Out"=w374:string)  [unwired: 13 in]
      }
    }
  }
  "error out" <- w2
